vi "GetMeasurementCurrentLimitRegister.vi"(8 "Error In":errorcluster, 10 "Register":T1(ring), 11 "Kiethley 2602 In":refnum<visa-resource-name>) -> (0 "Error Out":errorcluster, 2 "Measurement Current Limit Register":bool[](array[boolean]), 3 "Keithley 2602 Out":refnum<visa-resource-name>)   [LabVIEW 2012, in "Keithley-2602.lvlib"]
uses:
  Keithley-2602.lvlib
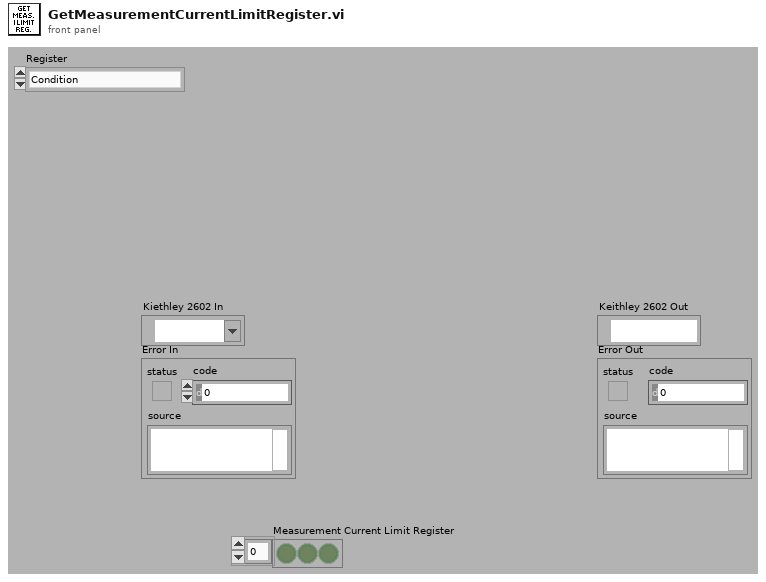
[diagram p1: front panel]
types:
  T1 = enum16{"Condition", "Event", "Enable", "Positive Transition", "Negative Transition"}
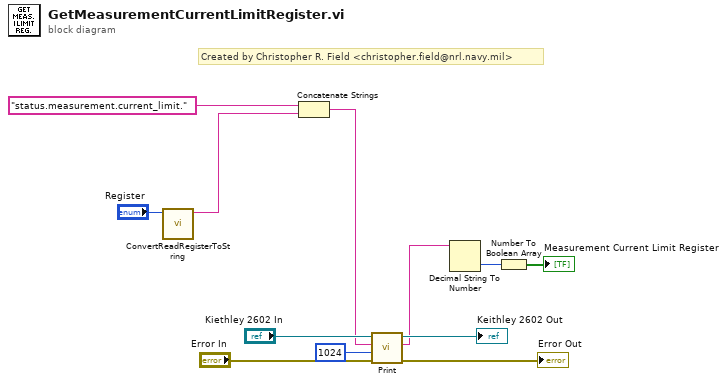
[diagram p0: block diagram]
diagram:
  # "Created by Christopher R. Field <christopher.field@nrl.navy.mil>"
  n1 = call "ConvertReadRegisterToString.vi"("Register"="Register") -> ("Register"=w2:string)  [unwired: 10 in]
  n2 = Concatenate Strings("status.measurement.current_limit.", w2) -> (w3:string)
  n3 = call "Print.vi"("Error In"="Error In", "Byte Count"=u32 1024, "Attribute"=w3, "Kiethley 2602 In"="Kiethley 2602 In") -> ("Error Out"=→"Error Out":errorcluster, "Output"=w7:string, "Keithley 2602 Out"=→"Keithley 2602 Out":refnum<visa-resource-name>)  [unwired: 5 in]
  n4 = Decimal String To Number(string=w7) -> (number=w6:i32)  [unwired: 2 in, 1 out]
  n5 = Number To Boolean Array(number=w6) -> (Boolean array=→"Measurement Current Limit Register":bool[])
